vi "Test Generate Mock Class Inherits from Source.vi"(8 "error in (no error)":errorcluster, 11 "Test Case In":refnum<class "Mock Class Generator Test.lvclass">) -> (0 "error out":errorcluster, 3 "Test Case Out":refnum<class "Mock Class Generator Test.lvclass">)   [LabVIEW 2020, in "Mock Class Generator Test.lvclass"]
uses:
  Mock Class Generator Test.lvclass
  C:/Program Files (x86)/National Instruments/LabVIEW 2020/vi.lib/Astemes/LUnit/Test Case.lvclass
  <vilib>/Astemes/LUnit/Test Case.lvclass/Test Case.ctl
  d61b9b24-4b0f-44ef-a9bb-4996cb077d5f.vi
  <vilib>/Astemes/LUnit/Append Pass Result.vi
  <vilib>/Astemes/LUnit/Append Fail Result.vi
  <vilib>/Astemes/LUnit/Describe Comparison.vi
  <vilib>/Astemes/LUnit/Compare Variants.vi
  <vilib>/Astemes/LUnit/Variant to string.vi
  <vilib>/Utility/Data Type/Get Type Information.vi
  <vilib>/Utility/LVClass/Get LV Class Name.vi
  source/Mock Class Generator/Mock Class Generator.lvclass
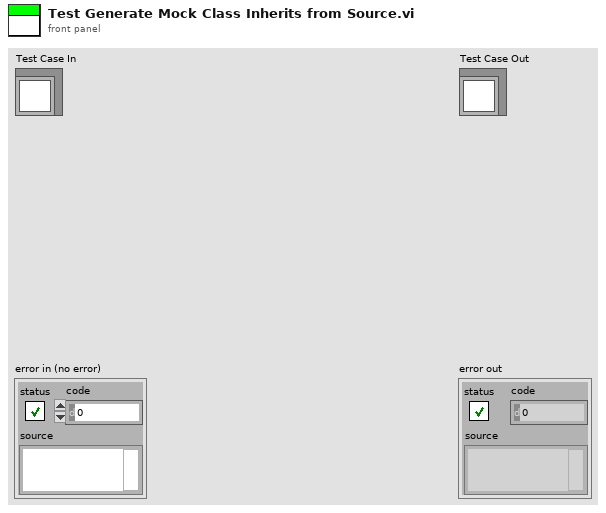
[diagram p1: front panel]
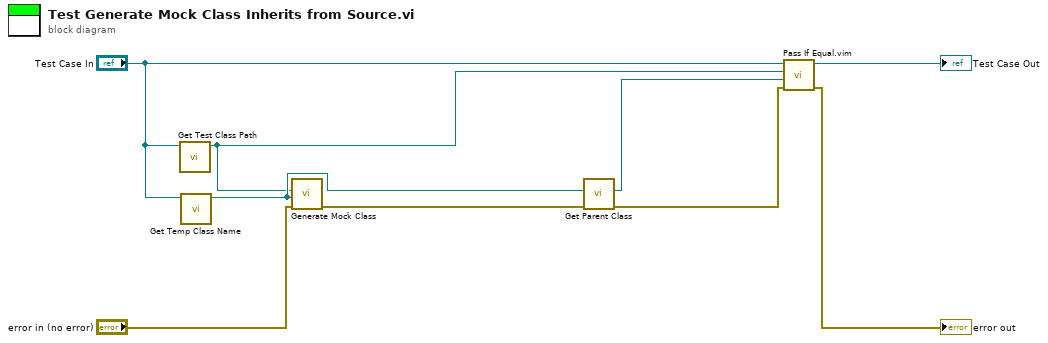
[diagram p0: block diagram]
diagram:
  n1 = call "Get Test Class Path.vi"("Mock Class Generator Test in"="Test Case In") -> ("Test Class Path"=w1:path)  [unwired: 10 in]
  n2 = call "Get Temp Class Name.vi"("Mock Class Generator Test in"="Test Case In") -> ("Test Class Path"=w5:path)  [unwired: 10 in]
  n3 = call "Generate Mock Class.vi"("error in (no error)"="error in (no error)", "Destination Class Path"=w5, "Source Class Path"=w1) -> ("error out"=w4:errorcluster)  [unwired: 8 in]
  n4 = call "Get Parent Class.vi"("error in (no error)"=w4, "Test Class Path"=w5) -> ("error out"=w3:errorcluster, "Path"=w2:path)  [unwired: 8 in]
  n5 = call "Pass If Equal.vim"("error in (no error)"=w3, "Actual"=w2, "Expected"=w1, "LUnit Test Case In"="Test Case In") -> ("error out"=→"error out":errorcluster, "LUnit Test Case Out"=→"Test Case Out":refnum<class "Mock Class Generator Test.lvclass">)  [unwired: 6 in]
